vi "NI-DP_AcknowledgeReply.vi"(5 "RX Port No.":u16, 6 "timeout [ms]":u32, 7 "IP to write to":string, 8 "error in (no error)":errorcluster, 11 "UDP Network Connection in":refnum<k16>) -> (0 "error out":errorcluster, 3 "UDP Network Connection out":refnum<k16>)   [LabVIEW 2014, in "hse-network.lvlib"]
doc: "____\nHAMPEL SOFTWARE ENGINEERING v0.7.0 (2018-07-16 18:12)"
uses:
  hse-network.lvlib
  NI-DP__Commands.ctl
  NI-DP__MessageStructure.ctl
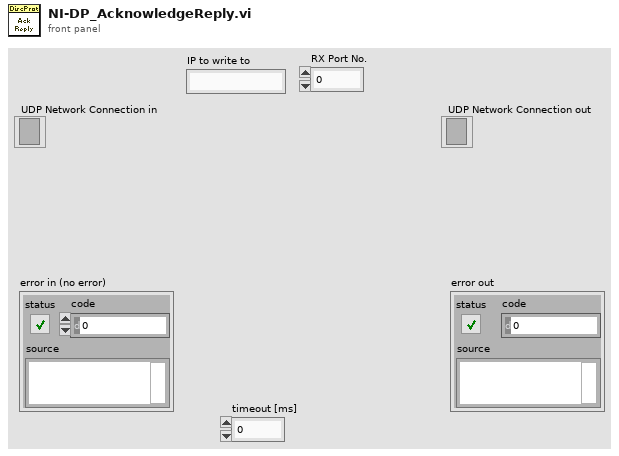
[diagram p1: front panel]
types:
  T1 = typedef "hse-network.lvlib/NI-DP__MessageStructure.ctl" = cluster{"Start of Message":string, "Command":T2, "Checksum(?) for P3,P4":string, "Always 0x02":string, "Model Code":string, "??? 1":string, "Serial":string, "Device Mac Address":string, "??? 2":string, "Param 1":string, "Param 2":string, "Param 3":string, "Param 4":string, "Checksum(?) for Network":string, "Device IP Address":string, "Device Subnet Mask":string, "Device DNS-Server":string, "Device Default Gateway":string, "??? 3":string, "End of Message":string}
  T2 = typedef "hse-network.lvlib/NI-DP__Commands.ctl" = u8
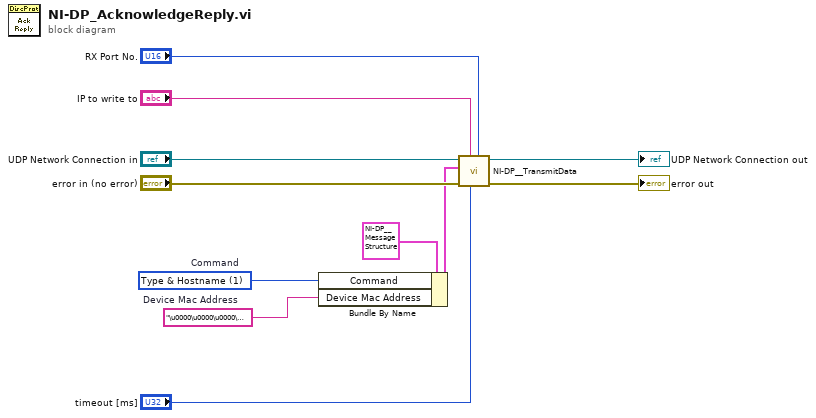
[diagram p0: block diagram]
diagram:
  w1 = "\u0000\u0000\u0000\u0000\u0000\u0000"  # Device Mac Address
  w2 = T2 1 items=["Type & Hostname"=1, "System State"=242, "Response"=32]  # Command
  n1 = Bundle By Name(cluster=T1 {"Start of Message"="ED", "Command"=1, "Checksum(?) for P3,P4"="\u0002", "Always 0x02"="\u0000\u0000\u0000\u0000\u0000\u0000\u0000\u0000", "Model Code"="\u0000\u0000\u0000\u0000\u0000\u0000\u0000\u0000", "??? 1"="\u0000\u0000", "Serial"="\u0000\u0000", "Device Mac Address"="\u0000\u0000\u0000\u0000\u0000\u0000", "??? 2"="\u0000\u0000\u0000\u0000\u0000\u0000\u0000\u0000\u0000\u0000\u0000\u0000\u0000\u0000\u0000\u0000", "Param 1"="", "Param 2"="", "Param 3"="\u0000\u0000\u0000\u0000\u0000\u0000\u0000\u0000\u0000\u0000\u0000\u0000\u0000\u0000\u0000\u0000\u0000\u0000\u0000\u0000\u0000\u0000\u0000\u0000\u0000\u0000\u0000\u0000\u0000\u0000\u0000\u0000", "Param 4"="\u0000\u0000\u0000\u0000\u0000\u0000\u0000\u0000\u0000\u0000\u0000\u0000\u0000\u0000\u0000\u0000\u0000\u0000\u0000\u0000\u0000\u0000\u0000\u0000\u0000\u0000\u0000\u0000\u0000\u0000\u0000\u0000", "Checksum(?) for Network"="\u0000\u0000", "Device IP Address"="\u0000\u0000\u0000\u0000", "Device Subnet Mask"="\u0000\u0000\u0000\u0000", "Device DNS-Server"="\u0000\u0000\u0000\u0000", "Device Default Gateway"="\u0000\u0000\u0000\u0000", "??? 3"="\u0000\u0000\u0000\u0000\u0000\u0000\u0000\u0000\u0000\u0000\u0000\u0000\u0000\u0000\u0000\u0000", "End of Message"="NI"} ("UDP-NI__SendData"), "Command"=w2, "Device Mac Address"=w1) -> (w3:T1)
  n2 = call "NI-DP__TransmitData.vi"("Port to write to"="RX Port No.", "timeout ms"="timeout [ms]", "IP to write to"="IP to write to", "error in"="error in (no error)", "UDP-NI__Message"=w3, "UDP Network Connection in"="UDP Network Connection in") -> ("error out"=→"error out":errorcluster, "UDP Network Connection out"=→"UDP Network Connection out":refnum<k16>)  [unwired: 4 in]
